vi "Configure IScan Trigger (Serial).vi"(0 "VISA resource name":refnum<visa-resource-name>, 5 "Channel (1: Channel1)":i32(ring)=1 items=["Channel1"=1, "Channel2"=2, "Channel3"=3, "Channel4"=4], 9 "Pattern (0)":string="0", 11 "error in (no error)":errorcluster) -> (4 "VISA resource name out":refnum<visa-resource-name>, 15 "error out":errorcluster)   [LabVIEW 2013, in "Agilent 90000 Series.lvlib"]
doc: "Configures InfiniiScan trigger under serial trigger mode."
uses:
  Agilent 90000 Series.lvlib
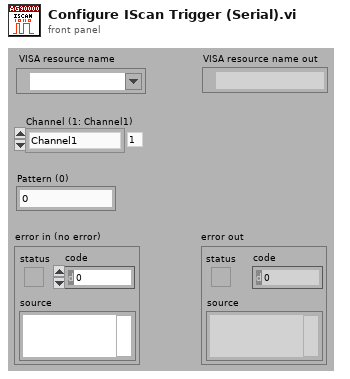
[diagram p1: front panel]
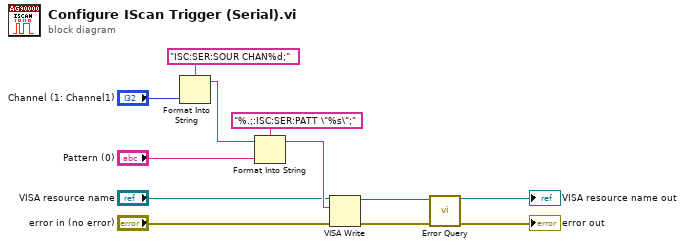
[diagram p0: block diagram]
diagram:
  n1 = Format Into String(format string="ISC:SER:SOUR CHAN%d;", "Channel (1: Channel1)") -> (resulting string=w10:string)  [unwired: 2 in, 1 out]
  n2 = Format Into String(format string="%.;:ISC:SER:PATT \"%s\";", initial string=w10, "Pattern (0)") -> (resulting string=w7:string)  [unwired: 1 in, 1 out]
  n3 = VISA Write(VISA resource name="VISA resource name", write buffer=w7, error in (no error)="error in (no error)") -> (VISA resource name out=w4:refnum<visa-resource-name>, error out=w3:errorcluster)  [unwired: 1 out]
  n4 = call "Error Query.vi"("error in (no error)"=w3, "VISA resource name"=w4) -> ("error out"=→"error out":errorcluster, "VISA resource name out"=→"VISA resource name out":refnum<visa-resource-name>)  [unwired: 8 out]
